vi "UserDefined.Compile.vi"(8 "error in (no error)":errorcluster, 11 "Section Ref in":T4 format="%.0x") -> (0 "error out":errorcluster, 2 "Settings":T1 {"Signal.Cmd.Refs"."Signal Refs" format="%.0x"; "Signal.Cmd.Info"."Signals"."Byte Order" items=["Little Endian", "Big Endian"]; "Signal.Cmd.Info"."Signals"."Data Type" items=["Signed", "Unsigned", "IEEE Float"]; "Settings.Refs"."Signal Refs" format="%.0x"; "Signal.Resp.Refs"."Signal Refs" format="%.0x"; "Signal.Resp.Info"."Signals"."Byte Order" items=["Little Endian", "Big Endian"]; "Signal.Resp.Info"."Signals"."Data Type" items=["Signed", "Unsigned", "IEEE Float"]; "Trigger.Refs"."Signal Refs" format="%.0x"; "Status.Refs"."Signal Refs" format="%.0x"}, 3 "Section Ref out":T4 format="%.0x")   [LabVIEW 2019, in "Diagnostics Addon System Explorer.lvlib"]
uses:
  Diagnostics Addon System Explorer.lvlib
  <vilib>/NI VeriStand/Custom Device API/Custom Device Item Ref.ctl
  Types/Service.Export.ctl
  Types/Frame.Ref.ctl
  Addon Shared/Types/Type.ctl
  Addon Shared/Types/Frame.Compile.ctl
  Addon Shared/Types/Signal.ctl
  Types/FG.Action.ctl
  Signal.FG.vi
  Frame.GetSignalRefs.vi
  Addon Shared/SubVIs/Constants.vi
  <vilib>/NI VeriStand/Custom Device Tools/Custom Device Utility Library/NI VeriStand - Search for All Items by GUID.vi
  <vilib>/NI VeriStand/Custom Device Tools/Custom Device Utility Library/NI VeriStand - Search for Item by GUID.vi
  <vilib>/NI VeriStand/Custom Device API/NI VeriStand - Get Item Children.vi
  <vilib>/NI VeriStand/Custom Device Tools/Custom Device Utility Library/NI VeriStand - Search for Item by Name.vi
  <vilib>/NI/NI VeriStand Advanced SysDef API/SysDef API/SysDef.Property.Set.vi
  <vilib>/NI/NI VeriStand Advanced SysDef API/_SubVIs/SysDef.Property.Set.U32.vi
  <vilib>/NI VeriStand/Custom Device API/NI VeriStand - Get Item Property.vi
  <vilib>/NI VeriStand/Custom Device API/Get Item Property (U32).vi
  <vilib>/NI VeriStand/Custom Device API/NI VeriStand - Get Item Data.vi
  <vilib>/NI/NI VeriStand Advanced SysDef API/_SubVIs/SysDef.Property.Set.DBL.vi
  <vilib>/NI/NI VeriStand Advanced SysDef API/_SubVIs/SysDef.Property.Set.String.vi
  <vilib>/NI VeriStand/Custom Device API/Get Item Property (Double).vi
  <vilib>/NI VeriStand/Custom Device API/Get Item Property (String).vi
  <vilib>/NI VeriStand/Custom Device API/NI VeriStand - Get Custom Device Channel Data.vi
  <vilib>/NI VeriStand/Custom Device Tools/Custom Device Utility Library/Custom Device Utility Library.lvlib
  <vilib>/NI VeriStand/Custom Device API/Custom Device API.lvlib
  Addon Shared/Diagnostics Addon Shared.lvlib
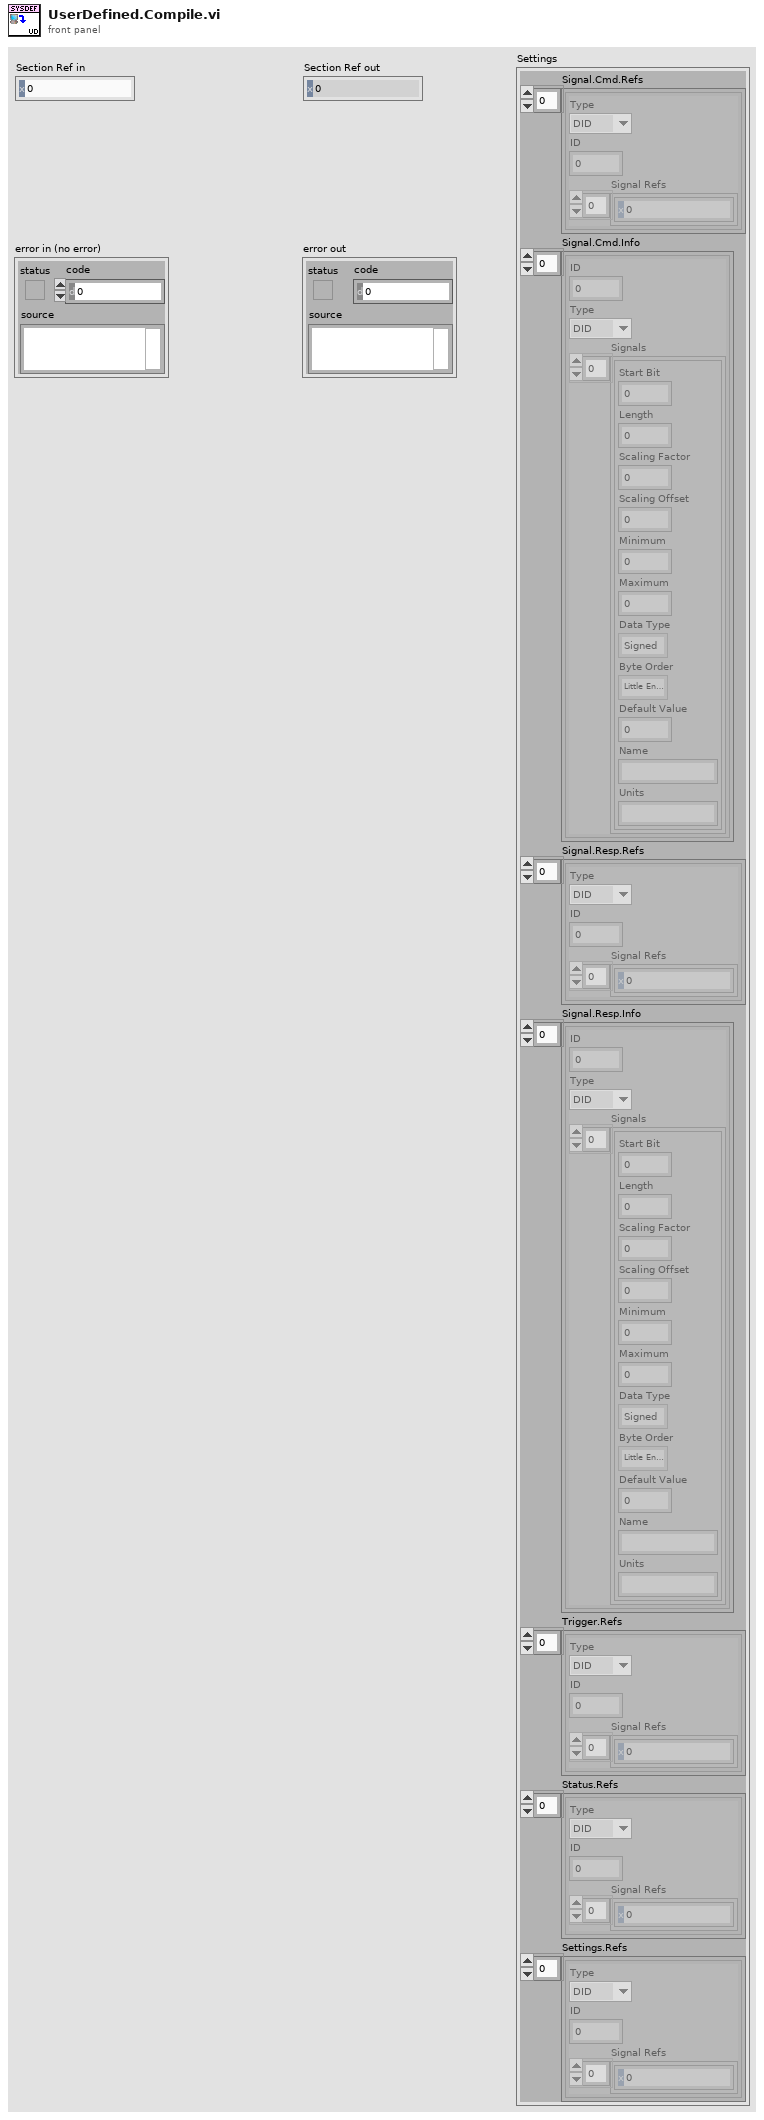
[diagram p1: front panel]
types:
  T1 = typedef "Diagnostics Addon System Explorer.lvlib/Service.Export.ctl" = cluster{"Signal.Cmd.Refs":T2[], "Signal.Cmd.Info":T5[], "Signal.Resp.Refs":T2[], "Signal.Resp.Info":T5[], "Trigger.Refs":T2[], "Status.Refs":T2[], "Settings.Refs":T2[]}
  T2 = typedef "Diagnostics Addon System Explorer.lvlib/Frame.Ref.ctl" = cluster{"Type":T3, "ID":u32, "Signal Refs":T4[]}
  T3 = typedef "Diagnostics Addon Shared.lvlib/Type.ctl" = enum16{"DID", "CDID", "PID", "CPID", "Read Memory", "Write Memory", "IO Control", "Routine Start", "Routine Request", "Routine Stop", "User Defined", "DTC Control", "Clear DTCs", "Read DTCs", "Start DTCs", "DTC Change Count", "Tester Present", "Unlock ECU", "Reset ECU", "Diag Session Control", "Communication Control", "DPID Control", "Poll Control", "Diag CAN Control"}
  T4 = typedef "Custom Device API.lvlib/Custom Device Item Ref.ctl" = u64
  T5 = typedef "Diagnostics Addon Shared.lvlib/Frame.Compile.ctl" = cluster{"ID":u32, "Type":T3, "Signals":T6[]}
  T6 = typedef "Diagnostics Addon Shared.lvlib/Signal.ctl" = cluster{"Start Bit":u32, "Length":u32, "Scaling Factor":dbl, "Scaling Offset":dbl, "Minimum":dbl, "Maximum":dbl, "Data Type":u32, "Byte Order":u32, "Default Value":dbl, "Name":string, "Units":string}
  T7 = typedef "Diagnostics Addon System Explorer.lvlib/FG.Action.ctl" = enum16{"Get", "Set"}
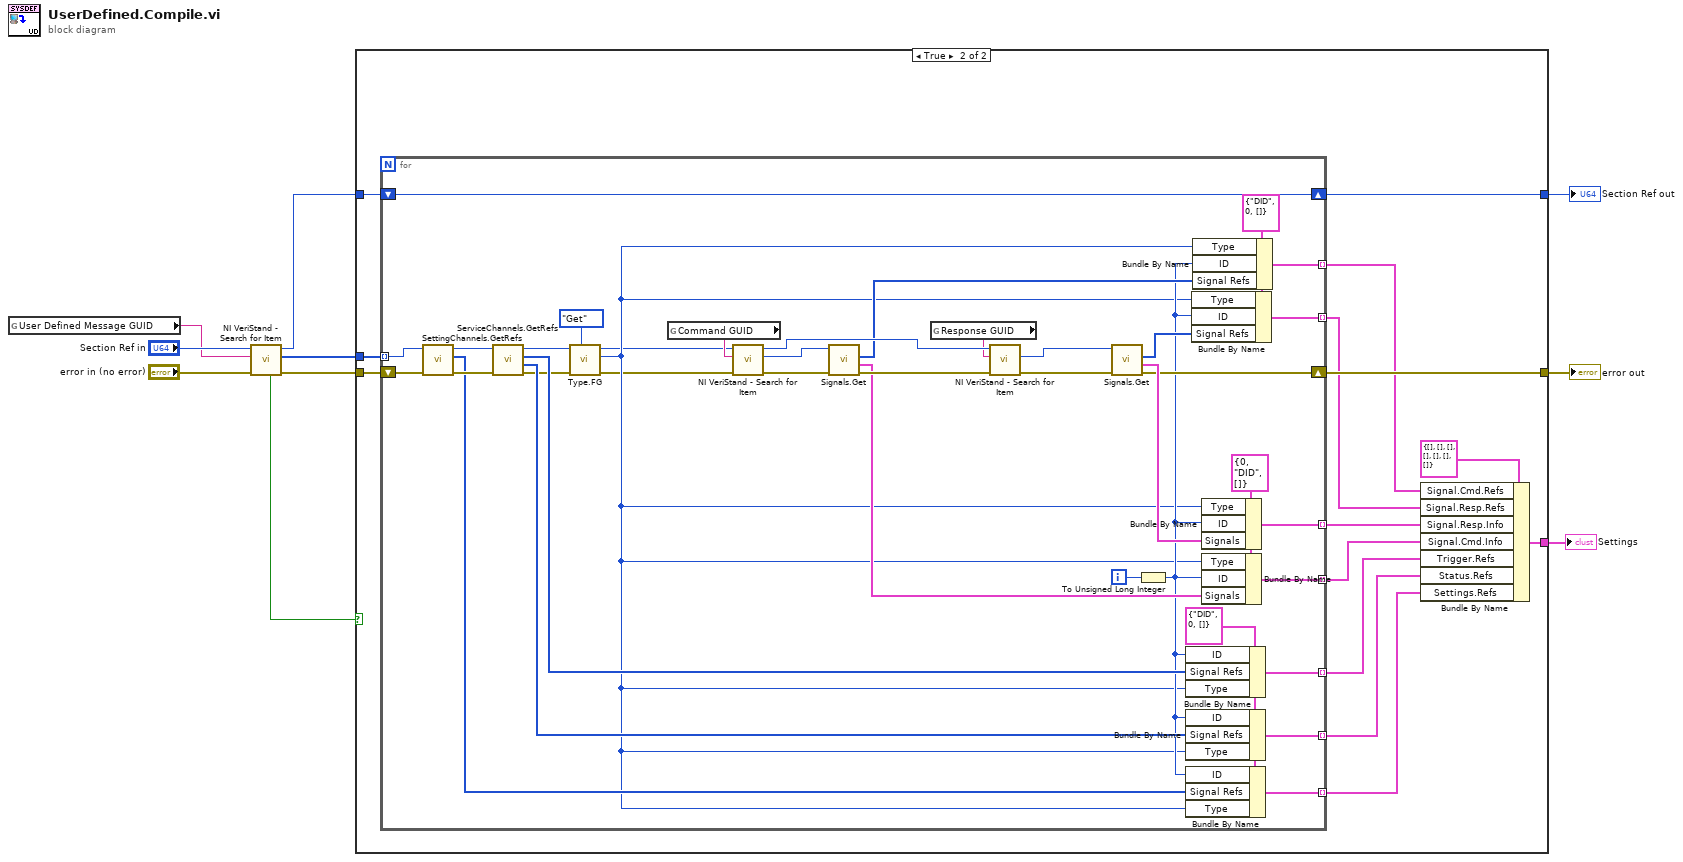
[diagram p0: block diagram]
diagram:
  n1 = global read "Constants.vi" "User Defined Message GUID"() -> (w4:string)
  n2 = call-poly <vilib>:"NI VeriStand - Search for Item.vi"("error in"="error in (no error)", "Item GUID"=w4, "Section Ref in"="Section Ref in") -> ("error out"=w6:errorcluster, "Item Refs"=w7:T4[], "Section Ref out"=w3:T4, "Found"=w5:bool)  [unwired: 5 in]
  n3 = case shown="True" w5 {
    tunnel: [w12 w26] -> w10
    tunnel: w7 -> [_ w24]
    tunnel: w6 -> [w12 w25]
    tunnel: w3 -> [w11 w23]
    tunnel: [w11 w22] -> w2
    tunnel: [_ w14] -> w1
    frame False {
    }
    frame True {
      n4 = for {
        shift-right: [w58] -> w26
        shift-left: w25 -> [w43]
        tunnel: w24 -> [w40] mode=indexing
        tunnel: [w57] -> w18 mode=indexing
        tunnel: [w56] -> w17 mode=indexing
        tunnel: [w52] -> w20 mode=indexing
        tunnel: [w51] -> w19 mode=indexing
        shift-right: [w49] -> w22
        shift-left: w23 -> [w49]
        tunnel: [w45] -> w16 mode=indexing
        tunnel: [w44] -> w15 mode=indexing
        tunnel: [w39] -> w13 mode=indexing
        i -> [w46]
        w38 = T2 {"Type"=enum."DID", "ID"=0, "Signal Refs"=[]} ("cluster")
        w54 = T2 {"Type"=enum."DID", "ID"=0, "Signal Refs"=[]} ("Cmd")
        w65 = T5 {"ID"=0, "Type"=enum."DID", "Signals"=[]} ("PID In")
        n5 = call "SettingChannels.GetRefs.vi"("error in (no error)"=w43, "Item Ref in"=w40) -> ("error out"=w42:errorcluster, "Settings"=w36:T4[], "Section Ref out"=w41:T4)  [unwired: 7 in]
        n6 = call "ServiceChannels.GetRefs.vi"("error in (no error)"=w42, "Item Ref in"=w41) -> ("error out"=w32:errorcluster, "Status"=w48:T4[], "Trigger"=w47:T4[], "Section Ref out"=w31:T4)  [unwired: 6 in]
        n7 = call "Type.FG.vi"("Action"=FG.Action."Get", "error in (no error)"=w32, "Device Item Ref in"=w31) -> ("error out"=w30:errorcluster, "Type"=w33:T3, "Device Item Ref out"=w29:T4)  [unwired: 6 in]
        n8 = global read "Constants.vi" "Command GUID"() -> (w61:string)
        n9 = call-poly <vilib>:"NI VeriStand - Search for Item.vi"("error in"=w30, "Item GUID"=w61, "Section Ref in"=w29) -> ("error out"=w28:errorcluster, "Item Ref"=w27:T4, "Section Ref out"=w63:T4)  [unwired: 5 in, 1 out]
        n10 = call "Signals.Get.vi"("error in (no error)"=w28, "Device Item Ref out"=w27) -> ("error out"=w64:errorcluster, "Parameters"=w60:T6[], "Child Refs"=w55:T4[])  [unwired: 6 in, 1 out]
        n11 = global read "Constants.vi" "Response GUID"() -> (w62:string)
        n12 = call-poly <vilib>:"NI VeriStand - Search for Item.vi"("error in"=w64, "Item GUID"=w62, "Section Ref in"=w63) -> ("error out"=w35:errorcluster, "Item Ref"=w34:T4)  [unwired: 5 in, 2 out]
        n13 = call "Signals.Get.vi"("error in (no error)"=w35, "Device Item Ref out"=w34) -> ("error out"=w58:errorcluster, "Parameters"=w59:T6[], "Child Refs"=w53:T4[])  [unwired: 6 in, 1 out]
        n14 = To Unsigned Long Integer(number=w46) -> (unsigned 32bit integer=w37:u32)
        n15 = Bundle By Name(cluster=w38, "ID"=w37, "Signal Refs"=w47, "Type"=w33) -> (w45:T2)
        n16 = Bundle By Name(cluster=w38, "ID"=w37, "Signal Refs"=w48, "Type"=w33) -> (w44:T2)
        n17 = Bundle By Name(cluster=w38, "ID"=w37, "Signal Refs"=w36, "Type"=w33) -> (w39:T2)
        n18 = Bundle By Name(cluster=w54, "Type"=w33, "ID"=w37, "Signal Refs"=w53) -> (w51:T2)
        n19 = Bundle By Name(cluster=w54, "Type"=w33, "ID"=w37, "Signal Refs"=w55) -> (w52:T2)
        n20 = Bundle By Name(cluster=w65, "Type"=w33, "ID"=w37, "Signals"=w59) -> (w57:T5)
        n21 = Bundle By Name(cluster=w65, "Type"=w33, "ID"=w37, "Signals"=w60) -> (w56:T5)
      }
      n22 = Bundle By Name(cluster=T1 {"Signal.Cmd.Refs"=[], "Signal.Cmd.Info"=[], "Signal.Resp.Refs"=[], "Signal.Resp.Info"=[], "Trigger.Refs"=[], "Status.Refs"=[], "Settings.Refs"=[]} ("Settings"), "Signal.Cmd.Refs"=w20, "Signal.Resp.Refs"=w19, "Signal.Resp.Info"=w18, "Signal.Cmd.Info"=w17, "Trigger.Refs"=w16, "Status.Refs"=w15, "Settings.Refs"=w13) -> (w14:T1)
    }
  }
  "Section Ref out" <- w2
  "error out" <- w10
  "Settings" <- w1
